vi "LOx_Weight.vi"() -> ()   [LabVIEW 2018]
panel:
  out "LOx Weight":dbl(knob) scale=0.0..150.0
  in  "End Loop":bool
  out "?":dbl
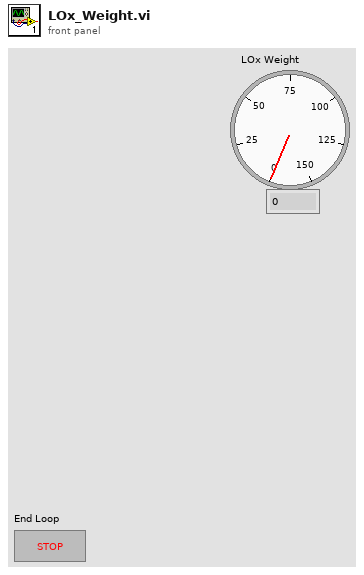
[diagram p1: front panel]
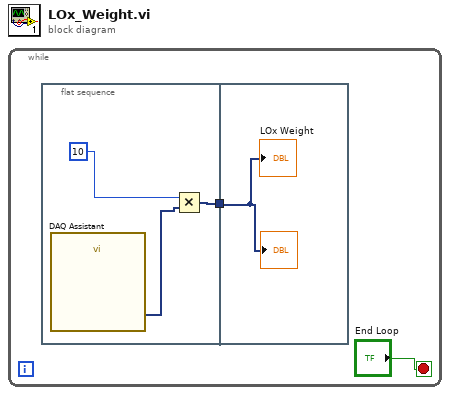
[diagram p0: block diagram]
diagram:
  n1 = while {
    stop <- "End Loop" stop-if-true
    n2 = flat-sequence {
      tunnel: [w4] -> w2
      tunnel: w2 -> [w6]
      frame #0 {
        n3 = call "DAQ Assistant"() -> ("data"=w3:dynamicdata)  [unwired: 17 in, 2 out]
        n4 = Multiply(x=10, y=w3) -> (x*y=w4:dynamicdata)
      }
      frame #1 {
        "?" <- w6
        "LOx Weight" <- w6
      }
    }
  }
